vi "Swerve_Module CanCoder Config.vi"(5 "Max # Of Tries":i32=5, 6 "Send Cmd Timout(ms)":u32=300, 7 "Specific Config Data":T2, 8 "Error":errorcluster, 9 "Module CanCoder Config Data":T4={"Direction Pos(t) Neg(f)"=TRUE}, 11 "CANcoder Ref":T1) -> (0 "Error Out":errorcluster, 3 "CANcoder Ref Out":T1)   [LabVIEW 2023]
uses:
  <vilib>/Rock Robotics/WPI/ThirdParty/Phoenix-LabVIEW/CANCoder/Controls/CTRE_Phoenix_CANcoder_SensorInitializationStrategy.ctl
  <vilib>/Rock Robotics/WPI/ThirdParty/Phoenix-LabVIEW/CANCoder/Controls/CTRE_Phoenix_CANcoder_AbsoluteSensorRange.ctl
  <vilib>/Utility/Data Type/NI_Data Type.lvlib
  <vilib>/Rock Robotics/WPI/ThirdParty/Phoenix-LabVIEW/CANCoder/Set/CTRE_Phoenix_CANcoder_SetPositionToAbsolute.vi
  <vilib>/Rock Robotics/WPI/ThirdParty/Phoenix-LabVIEW/CANCoder/Controls/CTRE_Phoenix_CANcoder_DeviceRef.ctl
  Shared Code/TypeDefs/ENUM_Motor Index.ctl
  Shared Code/TypeDefs/Cluster_Module Specific Config Data.ctl
  Shared Code/TypeDefs/Cluster_Swerve CanCoder Config Data.ctl
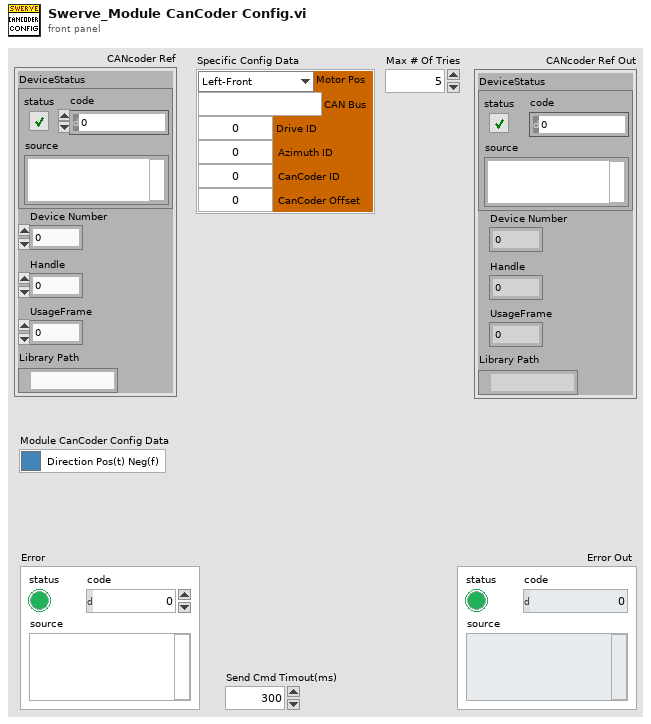
[diagram p1: front panel]
types:
  T1 = typedef "CTRE_Phoenix_CANcoder_DeviceRef.ctl" = cluster{"DeviceStatus":errorcluster, "Device Number":u8, "Handle":u64, "UsageFrame":u32, "Library Path":path}
  T2 = typedef "Cluster_Module Specific Config Data.ctl" = cluster{"Motor Pos":T3, "CAN Bus":string, "Drive ID":u8, "Azimuth ID":u8, "CanCoder ID":u8, "CanCoder Offset":dbl}
  T3 = typedef "ENUM_Motor Index.ctl" = enum16{"Left-Front", "Right-Front", "Left-Back", "Right-Back"}
  T4 = typedef "Cluster_Swerve CanCoder Config Data.ctl" = cluster{"Direction Pos(t) Neg(f)":bool}
  T5 = typedef "CTRE_Phoenix_CANcoder_SensorInitializationStrategy.ctl" = enum16{"Boot To Zero", "Boot To Absolute Position"}
  T6 = typedef "CTRE_Phoenix_CANcoder_AbsoluteSensorRange.ctl" = enum16{"Unsigned [0 to 360)", "Signed [-180 to +180)"}
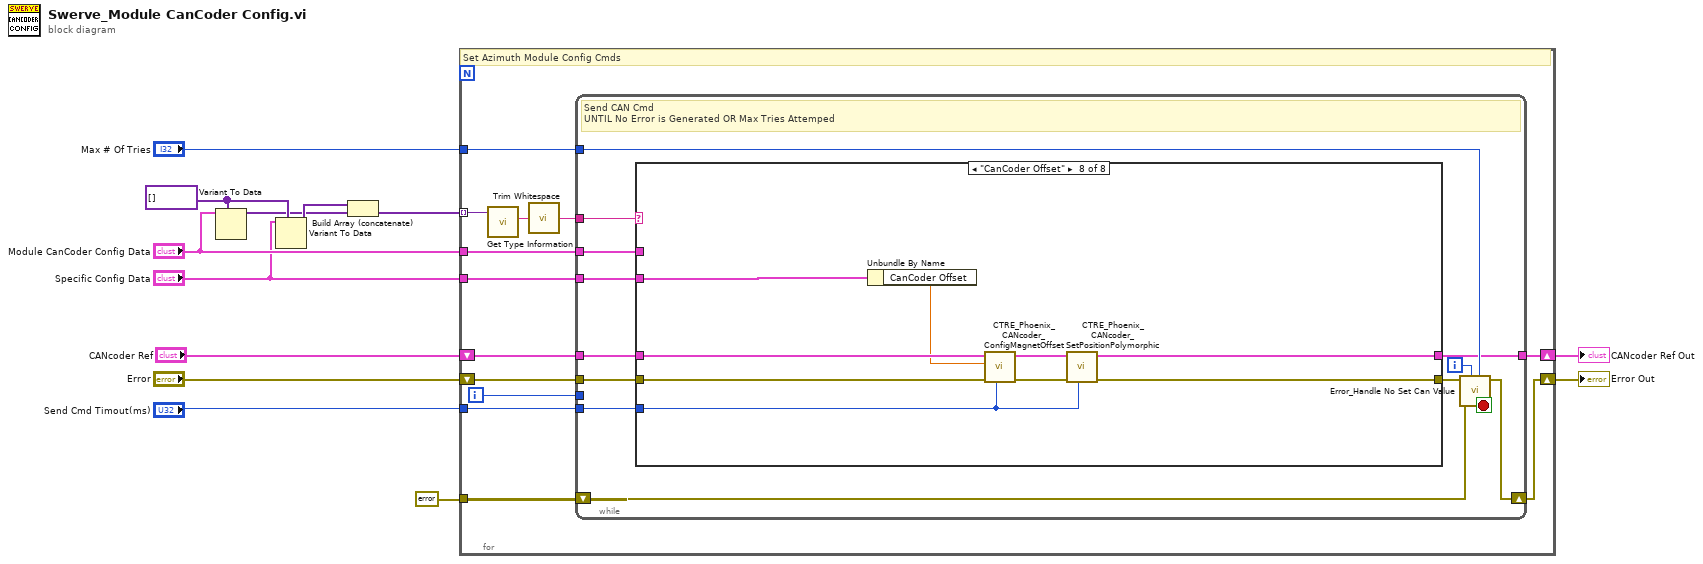
[diagram p0: block diagram]
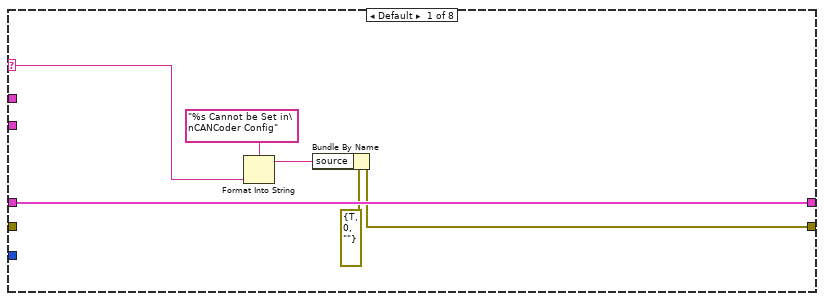
[diagram p2: hidden frame]
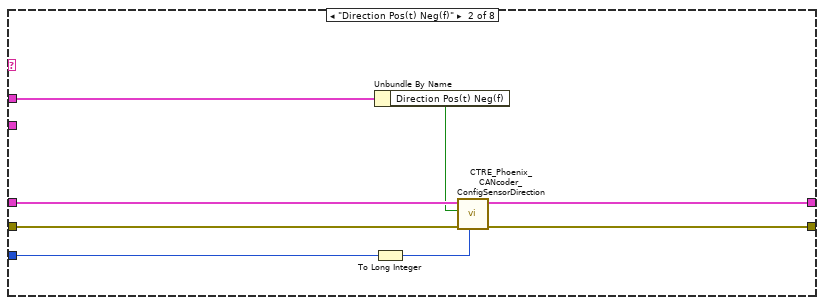
[diagram p3: hidden frame]
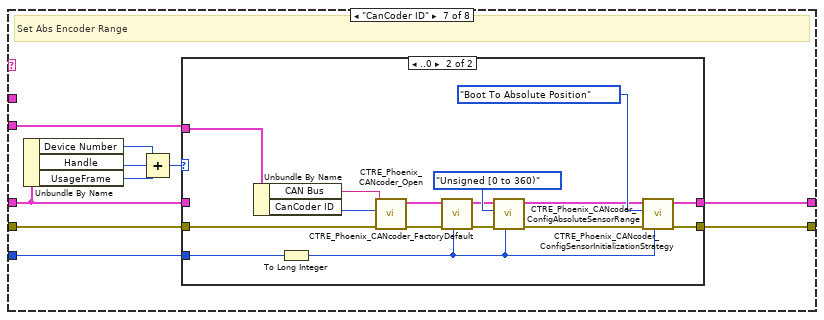
[diagram p8: hidden frame]
diagram:
  w5 = variant[] [] ("type")
  n1 = Variant To Data(type=w5, Variant="Module CanCoder Config Data") -> (data=w3:variant[])  [unwired: 1 in, 1 out]
  n2 = Variant To Data(type=w5, Variant="Specific Config Data") -> (data=w4:variant[])  [unwired: 1 in, 1 out]
  n3 = Build Array (concatenate)(w4, w3) -> (w2:variant[])
  n4 = for {
    tunnel: errorcluster {"status"=FALSE, "code"=0, "source"=""} ("Error Out") -> [w23]
    shift-right: [w25] -> w13
    shift-left: "Error" -> [w21]
    shift-right: [w26] -> w11
    shift-left: "CANcoder Ref" -> [w22]
    tunnel: "Module CanCoder Config Data" -> [w24]
    tunnel: "Max # Of Tries" -> [w19]
    tunnel: w2 -> [w17] mode=indexing
    tunnel: "Send Cmd Timout(ms)" -> [w15]
    tunnel: "Specific Config Data" -> [w14]
    i -> [w20]
    # "Set Azimuth Module Config Cmds"
    n5 = call <vilib>:"Get Type Information.vi"("variant"=w17) -> ("name"=w18:string)  [unwired: 6 in, 4 out]
    n6 = call <vilib>:"Trim Whitespace.vi"("string"=w18) -> ("trimmed string"=w16:string)  [unwired: 1 in]
    n7 = while {
      tunnel: [w29] -> w26
      tunnel: w15 -> [w36]
      shift-right: [w38] -> w25
      shift-left: w23 -> [w35]
      tunnel: w21 -> [w33]
      tunnel: w22 -> [w32]
      tunnel: w20 -> [_]
      tunnel: w24 -> [w31]
      tunnel: w19 -> [w30]
      tunnel: w16 -> [w28]
      tunnel: w14 -> [w27]
      i -> [w34]
      stop <- w37 stop-if-true
      # "Send CAN Cmd\nUNTIL No Error is Generated OR Max Tries Attemped"
      n8 = case shown="\"CanCoder Offset\"" w28 {
        selector: w28 -> [w43 _ _ _ _ _ _ _]
        tunnel: [w40 w51 w54 w56 w58 w61 w70 w91] -> w39
        tunnel: w36 -> [_ w49 _ _ _ _ w69 w93]
        tunnel: w33 -> [_ w50 w54 w56 w58 w61 w71 w92]
        tunnel: w32 -> [w42 w53 w55 w57 w59 w60 w62 w97]
        tunnel: w31 -> [_ w48 _ _ _ _ _ _]
        tunnel: [w42 w52 w55 w57 w59 w60 w68 w95] -> w29
        tunnel: w27 -> [_ _ _ _ _ _ w67 w90]
        frame Default {
          n9 = Format Into String(format string="%s Cannot be Set in\nCANCoder Config", w43) -> (resulting string=w44:string)  [unwired: 2 in, 1 out]
          n10 = Bundle By Name(cluster=errorcluster {"status"=TRUE, "code"=0, "source"=""} ("error out"), "source"=w44) -> (w40:errorcluster)
        }
        frame "Direction Pos(t) Neg(f)" {
          n11 = Unbundle By Name(w48) -> ("Direction Pos(t) Neg(f)"=w47:bool)
          n12 = To Long Integer(number=w49) -> (32bit integer=w46:i32)
          n13 = call <vilib>:"CTRE_Phoenix_CANcoder_ConfigSensorDirection.vi"("timeoutMs"=w46, "error in"=w50, "Sensor Direction"=w47, "CTRE_CANcoder_DeviceRef"=w53) -> ("error out"=w51:errorcluster, "CTRE_CANcoder_DeviceRef"=w52:T1)  [unwired: 6 in]
        }
        frame "Motor Pos" {
        }
        frame "CAN Bus" {
        }
        frame "Drive ID" {
        }
        frame "Azimuth ID" {
        }
        frame "CanCoder ID" {
          # "Set Abs Encoder Range"
          n14 = Unbundle By Name(w62) -> ("Device Number"=w65:u8, "Handle"=w66:u64, "UsageFrame"=w64:u32)
          n15 = Compound Arithmetic op=ADD(w65, w66, w64) -> (w63:u64)
          n16 = case shown="..0" w63 {
            tunnel: w71 -> [w73 w88]
            tunnel: [w73 w80] -> w70
            tunnel: w69 -> [_ w79]
            tunnel: [w72 w77] -> w68
            tunnel: w67 -> [_ w75]
            tunnel: w62 -> [w72 _]
            frame 1.. {
            }
            frame ..0 {
              n17 = Unbundle By Name(w75) -> ("CAN Bus"=w74:string, "CanCoder ID"=w87:u8)
              n18 = To Long Integer(number=w79) -> (32bit integer=w76:i32)
              n19 = call <vilib>:"CTRE_Phoenix_CANcoder_Open.vi"("error in"=w88, "Device Number"=w87, "CAN Bus"=w74) -> ("error out"=w84:errorcluster, "CTRE_CANcoder_DeviceRef"=w86:T1)  [unwired: 7 in]
              n20 = call <vilib>:"CTRE_Phoenix_CANcoder_FactoryDefault.vi"("timeoutMs"=w76, "error in"=w84, "CTRE_CANcoder_DeviceRef"=w86) -> ("error out"=w83:errorcluster, "CTRE_CANcoder_DeviceRef"=w85:T1)  [unwired: 7 in]
              n21 = call <vilib>:"CTRE_Phoenix_CANcoder_ConfigAbsoluteSensorRange.vi"("timeoutMs"=w76, "error in"=w83, "Absolute Sensor Range"=CTRE_Phoenix_CANcoder_AbsoluteSensorRange."Unsigned [0 to 360)", "CTRE_CANcoder_DeviceRef"=w85) -> ("error out"=w81:errorcluster, "CTRE_CANcoder_DeviceRef"=w78:T1)  [unwired: 6 in]
              n22 = call <vilib>:"CTRE_Phoenix_CANcoder_ConfigSensorInitializationStrategy.vi"("timeoutMs"=w76, "error in"=w81, "Sensor Initialization Strategy"=CTRE_Phoenix_CANcoder_SensorInitializationStrategy."Boot To Absolute Position", "CTRE_CANcoder_DeviceRef"=w78) -> ("error out"=w80:errorcluster, "CTRE_CANcoder_DeviceRef"=w77:T1)  [unwired: 6 in]
            }
          }
        }
        frame "CanCoder Offset" {
          n23 = Unbundle By Name(w90) -> ("CanCoder Offset"=w96:dbl)
          n24 = call <vilib>:"CTRE_Phoenix_CANcoder_ConfigMagnetOffset.vi"("timeoutMs"=w93, "error in"=w92, "Magnet Offset (Degrees)"=w96, "CTRE_CANcoder_DeviceRef"=w97) -> ("error out"=w94:errorcluster, "CTRE_CANcoder_DeviceRef"=w98:T1)  [unwired: 6 in]
          n25 = call-poly <vilib>:"CTRE_Phoenix_CANcoder_SetPositionPolymorphic.vi"("timeoutMs"=w93, "error in (no error)"=w94, "CTRE_CANcoder_DeviceRef"=w98) -> ("error out"=w91:errorcluster, "CTRE_CANcoder_DeviceRef"=w95:T1)  [unwired: 7 in]
        }
      }
      n26 = call "Error_Handle No Set Can Value.vi"("Max # Of Tries"=w30, "Loop Itteration"=w34, "Previous Error"=w35, "Error"=w39) -> ("Stop Out"=w37:bool, "Error Out"=w38:errorcluster)  [unwired: 6 in]
    }
  }
  "Error Out" <- w13
  "CANcoder Ref Out" <- w11
